vi "Error Magnitude.vi"(10 "Actual Task Coordinates (cm)":dbl[](array[numeric]), 11 "Desired Task Coordinates (cm)":dbl[](array[numeric])) -> (3 "Task-space\nError":dbl)   [LabVIEW 2018]
uses:
  <vilib>/Analysis/baseanly.llb/Real Dot Product.vi
  <vilib>/Analysis/NI_AALBase.lvlib
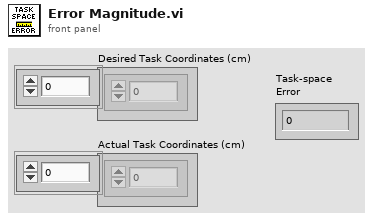
[diagram p1: front panel]
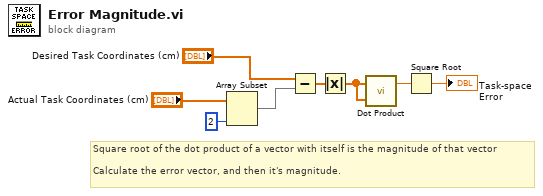
[diagram p0: block diagram]
diagram:
  # "Square root of the dot product of a vector with itself is the magnitude of that vector\n\nCalculate the error vector, and then it's magnitude."
  n1 = Array Subset(array="Actual Task Coordinates (cm)", length=2) -> (w1:dbl[])  [unwired: 1 in]
  n2 = Subtract(x="Desired Task Coordinates (cm)", y=w1) -> (x-y=w5:dbl[])
  n3 = Absolute Value(x=w5) -> (abs(x)=w6:dbl[])
  n4 = call-poly <vilib>:"Dot Product.vi"("Y Vector"=w6, "X Vector"=w6) -> ("X * Y"=w7:dbl)  [unwired: 1 out]
  n5 = Square Root(x=w7) -> (sqrt(x)=→"Task-space\nError":dbl)
